vi "Etalon Scan Routine.vi"() -> ()   [LabVIEW 2013]
uses:
  Agilis Control/Type Definitions/Etalon Scanner States.ctl
  Agilis Control/Type Definitions/Movement Direction.ctl
panel:
  in  "step size":i32=100
  in  "thick left limit":dbl
  in  "thick right limit":dbl
  in  "upper limit thin":dbl=1500.0
  out "Thick Acq":dbl
  out "Thin Acq":dbl
  out "Thick Setpoint":dbl
  out "Thin Setpoint":dbl
  in  "stepping interval (ms)":u32=200
  out "Array":cluster{"X Position":i32, "Y Position":i32}[](array[cluster])
  out "Loop Counter":i32
  in  "Stop":bool
  out "XY Position Graph":T1(graph)
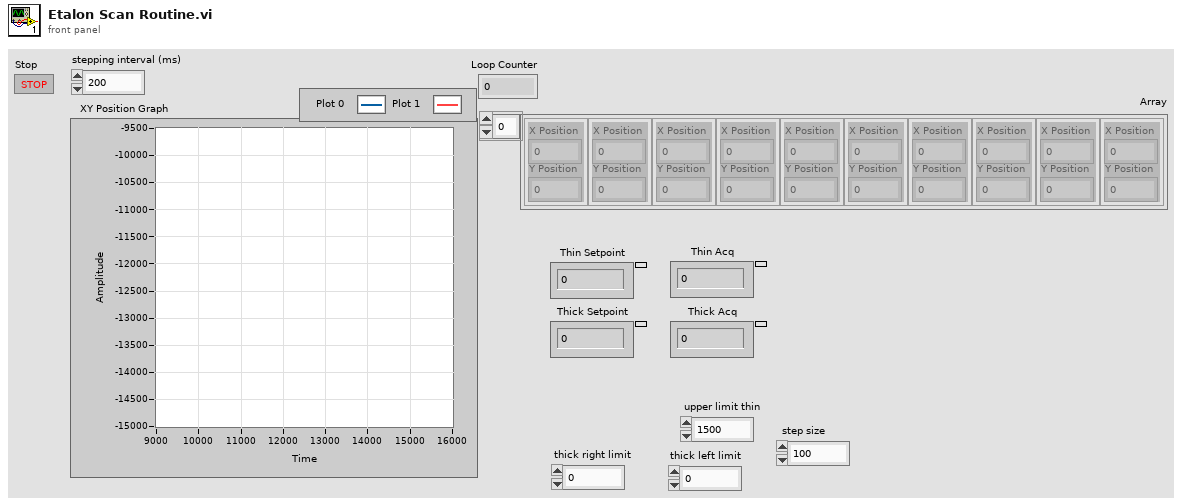
[diagram p1: front panel]
types:
  T1 = cluster{cluster{"Thin Acq":dbl, "Thick Acq":dbl}[]}[]
  T2 = typedef "Movement Direction.ctl" = enum16{"Left", "Right"}
  T3 = typedef "Etalon Scanner States.ctl" = enum16{"Idle", "Initialize", "Reset", "Go to Start", "Go Up", "Go Right", "Go Left", "Check Limit", "Move from Limit", "Shutdown"}
  T4 = cluster{cluster{"Thick Acq":dbl, "Thin Acq":dbl}[]}
  T5 = cluster{cluster{"Thick Acq":dbl, "Thin Acq":dbl}[]}[]
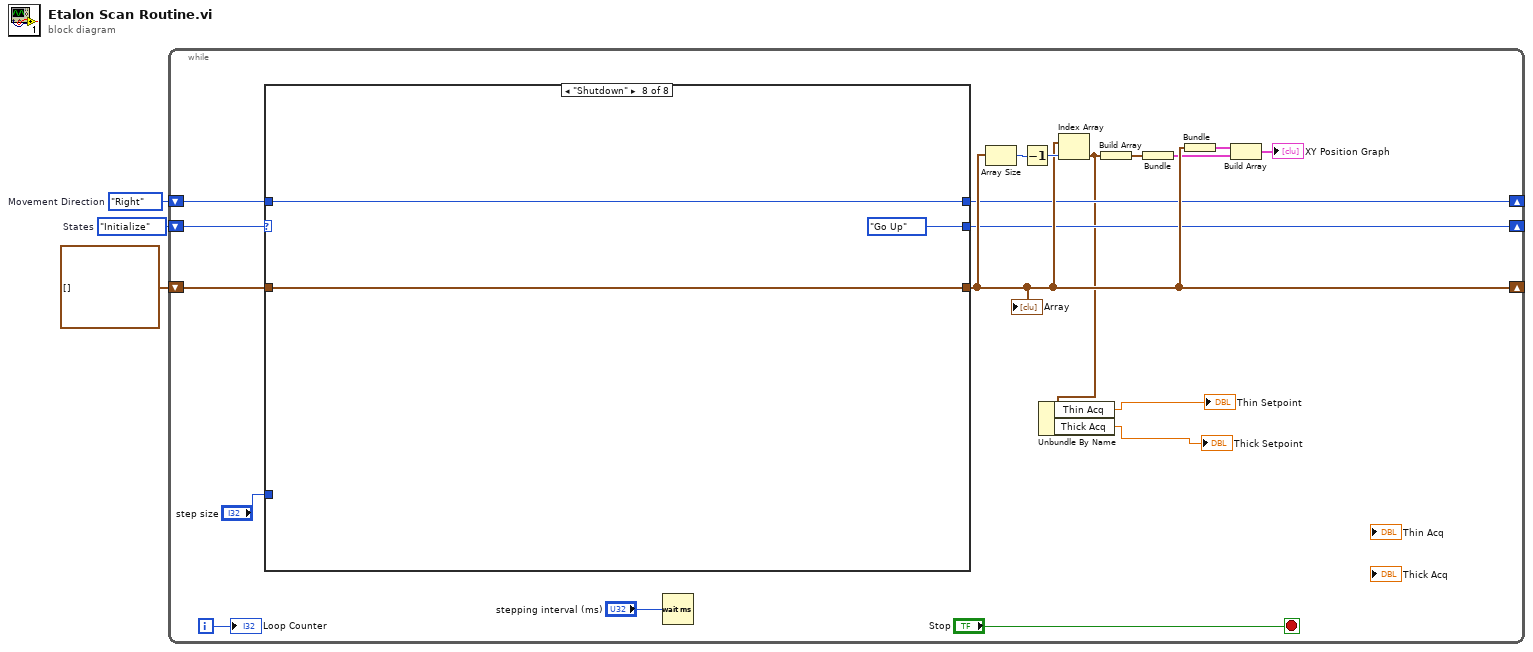
[diagram p0: block diagram]
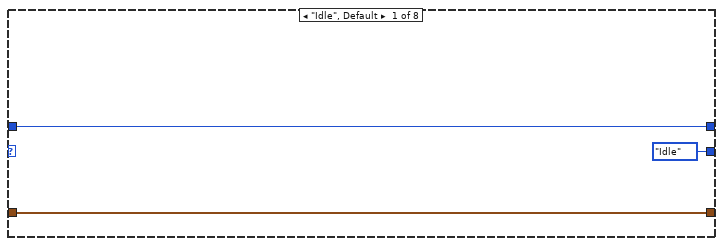
[diagram p2: hidden frame]
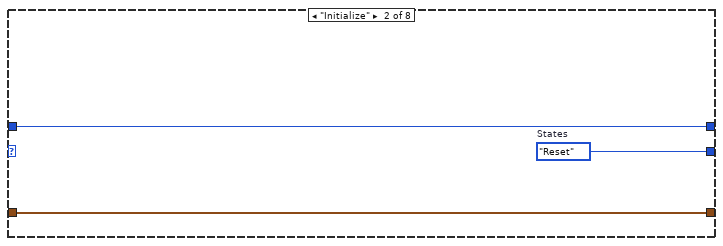
[diagram p3: hidden frame]
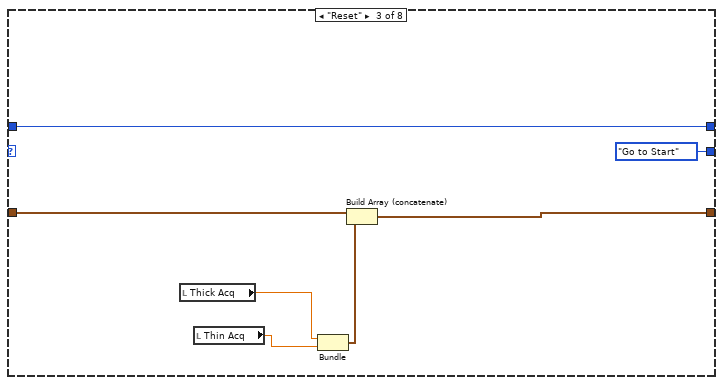
[diagram p4: hidden frame]
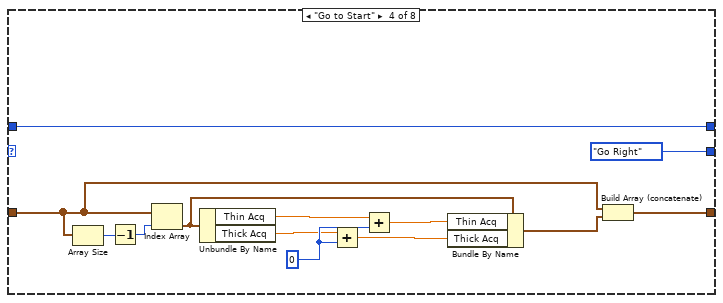
[diagram p5: hidden frame]
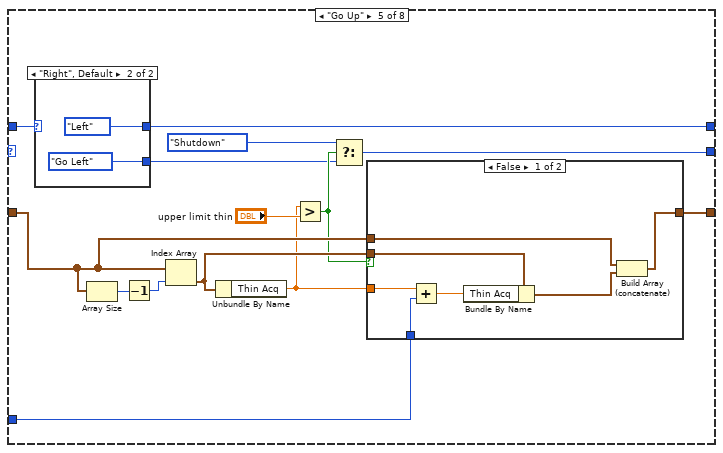
[diagram p6: hidden frame]
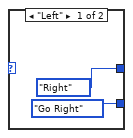
[diagram p7: hidden frame]
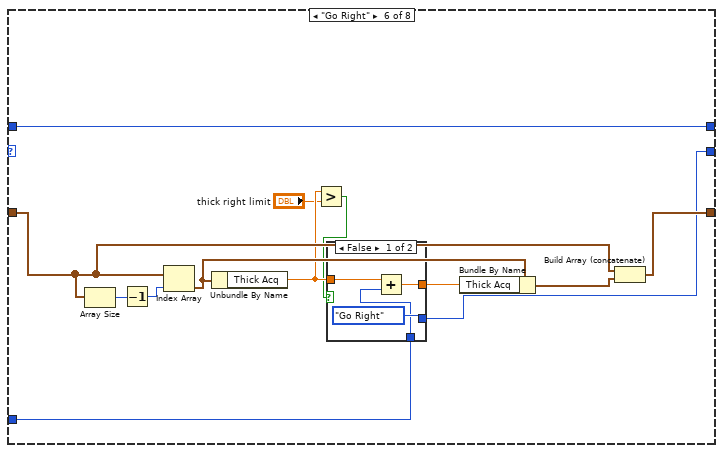
[diagram p9: hidden frame]
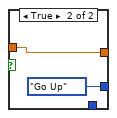
[diagram p10: hidden frame]
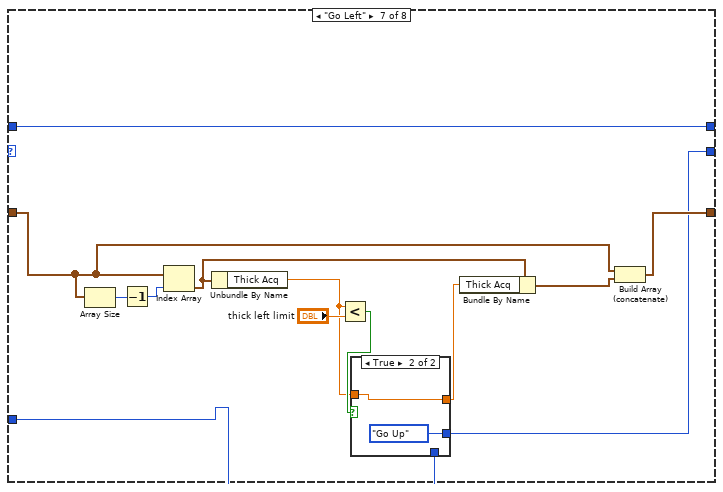
[diagram p11: hidden frame]
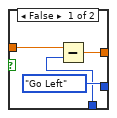
[diagram p12: hidden frame]
diagram:
  w2 = Movement_Direction."Right"  # Movement Direction
  w3 = Etalon_Scanner_States."Initialize"  # States
  n1 = while {
    shift-right: [w15] -> _
    shift-left: cluster{"Thick Acq":dbl, "Thin Acq":dbl}[] [] -> [w19]
    shift-right: [w8] -> _
    shift-left: w3 -> [w20]
    shift-right: [w9] -> _
    shift-left: w2 -> [w10]
    i -> [w21]
    stop <- "Stop" stop-if-true
    n2 = case shown="\"Shutdown\"" w20 {
      tunnel: w19 -> [w25 w28 w34 w41 w59 w82 w102 w115]
      tunnel: [w25 w28 w35 w39 w58 w81 w101 w115] -> w15
      tunnel: [Etalon_Scanner_States."Idle" ("States") w27 Etalon_Scanner_States."Go to Start" ("States") Etalon_Scanner_States."Go Right" ("States") w55 w76 w94 Etalon_Scanner_States."Go Up" ("States")] -> w8
      tunnel: w10 -> [w23 w26 w32 w36 w52 w80 w100 w113]
      tunnel: [w23 w26 w32 w36 w50 w80 w100 w113] -> w9
      tunnel: "step size" -> [_ _ _ _ w49 w75 w95 _]
      frame "Idle", Default {
      }
      frame "Initialize" {
        w27 = Etalon_Scanner_States."Reset"  # States
      }
      frame "Reset" {
        n3 = local read "Thick Acq"() -> (w29:dbl)
        n4 = local read "Thin Acq"() -> (w30:dbl)
        n5 = Bundle("Thick Acq"=w29, "Thin Acq"=w30) -> (w31:cluster{"Thick Acq":dbl, "Thin Acq":dbl})  [unwired: 1 in]
        n6 = Build Array (concatenate)(w34, w31) -> (w35:cluster{"Thick Acq":dbl, "Thin Acq":dbl}[])
      }
      frame "Go to Start" {
        w46 = 0
        n7 = Array Size(array=w41) -> (size(s)=w48:i32)
        n8 = Decrement(x=w48) -> (x-1=w47:i32)
        n9 = Index Array(array=w41, index=w47) -> (element=w38:cluster{"Thick Acq":dbl, "Thin Acq":dbl})
        n10 = Unbundle By Name(w38) -> ("Thin Acq"=w45:dbl, "Thick Acq"=w44:dbl)
        n11 = Add(x=w44, y=w46) -> (x+y=w42:dbl)
        n12 = Add(x=w45, y=w46) -> (x+y=w43:dbl)
        n13 = Bundle By Name(cluster=w38, "Thin Acq"=w43, "Thick Acq"=w42) -> (w40:cluster{"Thick Acq":dbl, "Thin Acq":dbl})
        n14 = Build Array (concatenate)(w41, w40) -> (w39:cluster{"Thick Acq":dbl, "Thin Acq":dbl}[])
      }
      frame "Go Up" {
        n15 = case shown="\"Right\", Default" w52 {
          tunnel: [Etalon_Scanner_States."Go Right" ("States") Etalon_Scanner_States."Go Left" ("States")] -> w51
          tunnel: [Movement_Direction."Right" Movement_Direction."Left"] -> w50
          frame "Left" {
          }
          frame "Right", Default {
          }
        }
        n16 = Array Size(array=w59) -> (size(s)=w62:i32)
        n17 = Decrement(x=w62) -> (x-1=w61:i32)
        n18 = Index Array(array=w59, index=w61) -> (element=w60:cluster{"Thick Acq":dbl, "Thin Acq":dbl})
        n19 = Unbundle By Name(w60) -> ("Thin Acq"=w53:dbl)
        n20 = Greater?(x=w53, y="upper limit thin") -> (0:w54:bool)
        n21 = Select(t=Etalon_Scanner_States."Shutdown" ("States"), s=w54, f=w51) -> (s? t:f=w55:T3)
        n22 = case shown="False" w54 {
          tunnel: w60 -> [w72 _]
          tunnel: w59 -> [w71 w74]
          tunnel: [w70 w74] -> w58
          tunnel: w53 -> [w68 _]
          tunnel: w49 -> [w67 _]
          frame False {
            n23 = Add(x=w68, y=w67) -> (x+y=w69:dbl)
            n24 = Bundle By Name(cluster=w72, "Thin Acq"=w69) -> (w73:cluster{"Thick Acq":dbl, "Thin Acq":dbl})
            n25 = Build Array (concatenate)(w71, w73) -> (w70:cluster{"Thick Acq":dbl, "Thin Acq":dbl}[])
          }
          frame True {
          }
        }
      }
      frame "Go Right" {
        n26 = Array Size(array=w82) -> (size(s)=w87:i32)
        n27 = Decrement(x=w87) -> (x-1=w86:i32)
        n28 = Index Array(array=w82, index=w86) -> (element=w83:cluster{"Thick Acq":dbl, "Thin Acq":dbl})
        n29 = Unbundle By Name(w83) -> ("Thick Acq"=w79:dbl)
        n30 = Greater?(x=w79, y="thick right limit") -> (0:w77:bool)
        n31 = case shown="False" w77 {
          tunnel: [w91 w93] -> w85
          tunnel: w79 -> [w90 w93]
          tunnel: [Etalon_Scanner_States."Go Right" ("States") Etalon_Scanner_States."Go Up" ("States")] -> w76
          tunnel: w75 -> [w88 _]
          frame False {
            n32 = Add(x=w90, y=w88) -> (x+y=w91:dbl)
          }
          frame True {
          }
        }
        n33 = Bundle By Name(cluster=w83, "Thick Acq"=w85) -> (w84:cluster{"Thick Acq":dbl, "Thin Acq":dbl})
        n34 = Build Array (concatenate)(w82, w84) -> (w81:cluster{"Thick Acq":dbl, "Thin Acq":dbl}[])
      }
      frame "Go Left" {
        n35 = Array Size(array=w102) -> (size(s)=w106:i32)
        n36 = Decrement(x=w106) -> (x-1=w105:i32)
        n37 = Index Array(array=w102, index=w105) -> (element=w103:cluster{"Thick Acq":dbl, "Thin Acq":dbl})
        n38 = Unbundle By Name(w103) -> ("Thick Acq"=w97:dbl)
        n39 = Less?(x=w97, y="thick left limit") -> (x < y?=w98:bool)
        n40 = case shown="True" w98 {
          tunnel: [w110 w112] -> w96
          tunnel: w97 -> [w109 w112]
          tunnel: [Etalon_Scanner_States."Go Left" ("States") Etalon_Scanner_States."Go Up" ("States")] -> w94
          tunnel: w95 -> [w107 _]
          frame False {
            n41 = Subtract(x=w109, y=w107) -> (x-y=w110:dbl)
          }
          frame True {
          }
        }
        n42 = Bundle By Name(cluster=w103, "Thick Acq"=w96) -> (w104:cluster{"Thick Acq":dbl, "Thin Acq":dbl})
        n43 = Build Array (concatenate)(w102, w104) -> (w101:cluster{"Thick Acq":dbl, "Thin Acq":dbl}[])
      }
      frame "Shutdown" {
      }
    }
    "Array" <- w15
    n44 = Wait (ms)(milliseconds to wait="stepping interval (ms)") -> ()  [unwired: 1 out]
    n45 = Array Size(array=w15) -> (size(s)=w17:i32)
    n46 = Decrement(x=w17) -> (x-1=w16:i32)
    n47 = Index Array(array=w15, index=w16) -> (element=w7:cluster{"Thick Acq":dbl, "Thin Acq":dbl})
    n48 = Unbundle By Name(w7) -> ("Thin Acq"=→"Thin Setpoint":dbl, "Thick Acq"=→"Thick Setpoint":dbl)
    n49 = Build Array(w7) -> (w14:cluster{"Thick Acq":dbl, "Thin Acq":dbl}[])
    n50 = Bundle(w14) -> (w12:T4)  [unwired: 1 in]
    n51 = Bundle(w15) -> (w13:T4)  [unwired: 1 in]
    n52 = Build Array(w13, w12) -> (→"XY Position Graph":T5)
    "Loop Counter" <- w21
  }
